vi "State_Machine.vi"(8 "error in (no error)":errorcluster caption="entrée d'erreur (pas d'erreur)", 11 "Get_Voltage en entrée":refnum<class "P2056_Get_SN.lvclass">) -> (0 "error out":errorcluster caption="sortie d'erreur", 2 "Json_String":string, 3 "Get_Voltage en sortie":refnum<class "P2056_Get_SN.lvclass">)   [LabVIEW 2020, in "Library Test.lvlib" / "P2056_Get_SN.lvclass"]
uses:
  P2056_Get_SN.lvclass
  C:/Users/ngarcin/OneDrive - Altyor/Standard TB/Class/Test/P2056_Send_Command_UART/P2056_Send_Command_UART.lvclass
  P2056_Send_Command_UART.lvclass
  P2056_Get_SN.lvclass/P2056_Get_SN.ctl
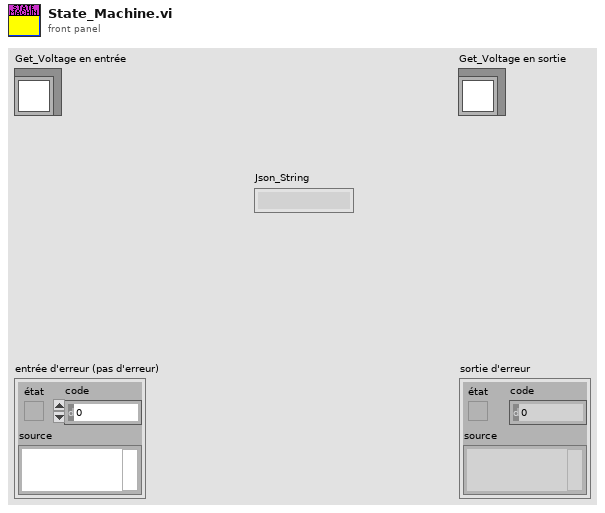
[diagram p1: front panel]
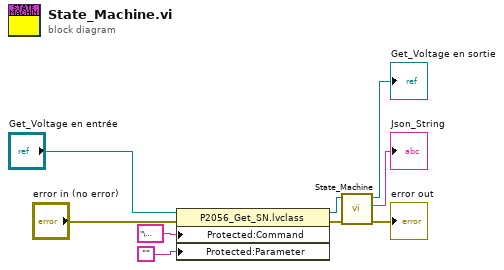
[diagram p0: block diagram]
diagram:
  n1 = property class="P2056_Get_SN.lvclass"(reference="Get_Voltage en entrée", error in="error in (no error)", "Protected:Command"="\u0016" ("chaîne"), "Protected:Parameter"="") -> (reference out=w7:refnum<class "P2056_Get_SN.lvclass">, error out=w6:errorcluster)
  n2 = call-parent "State_Machine.vi"("error in (no error)"=w6, "Get_Voltage en entrée"=w7) -> ("error out"=→"error out":errorcluster, "Json_String"=→"Json_String":string, "Get_Voltage en sortie"=→"Get_Voltage en sortie":refnum<class "P2056_Get_SN.lvclass">)  [unwired: 7 in]
